vi "rand_max.vi"(1 "Val_max":dbl) -> (0 "Val_out":dbl)   [LabVIEW 2009]
doc: "Generator de numere aleatoare setabil"
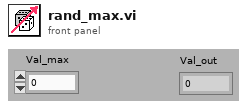
[diagram p1: front panel]
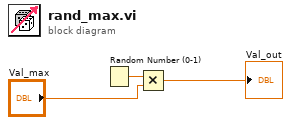
[diagram p0: block diagram]
diagram:
  n1 = Random Number (0-1)() -> (number: 0 to 1=w3:dbl)
  n2 = Multiply(x=w3, y="Val_max") -> (x*y=→"Val_out":dbl)
